vi "p33 operadoresf.vi"() -> ()   [LabVIEW 2017]
panel:
  in  "Enum 2":T1(ring)
  in  "path to BMP file":path
  in  "Tab Control":enum32{"Page 1"}(tab)
  out "2D Picture 15":picture
  out "2D Picture 16":picture
  in  "Slide 6":cluster{dbl, dbl, dbl, dbl, dbl}(slide)={0.0, 36.63140311804009, 185.40268456375838, 170.28523489932886, 152.88590604026845} scale=0.0..255.0
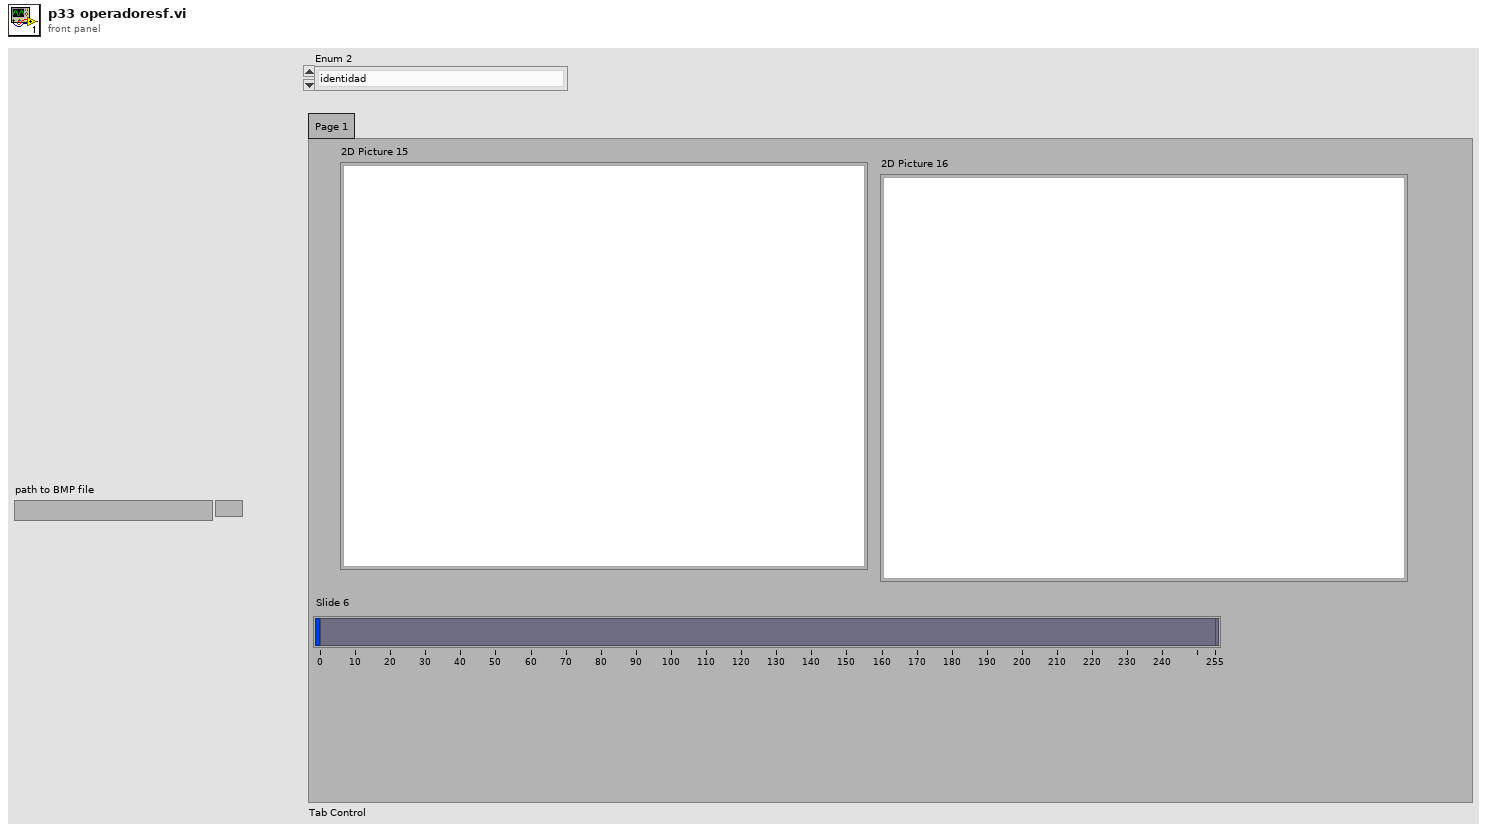
[diagram p1: front panel]
types:
  T1 = enum16{"identidad", "inverso o negativo", "umbral", "intervalo de umbral binario", "intervalo de umbral binario invertido", "umbral de la escala de grises", "umbral de la escala de grises invertido", "extension", "reduccion de nivel de gris", "ondulacion"}
  T2 = typedef "imagedata.ctl" = cluster{"image type":i32, "image depth":i32, "image":u8[], "mask":u8[], "colors":u32[], "Rectangle":cluster{"left":i16, "top":i16, "right":i16, "bottom":i16}}
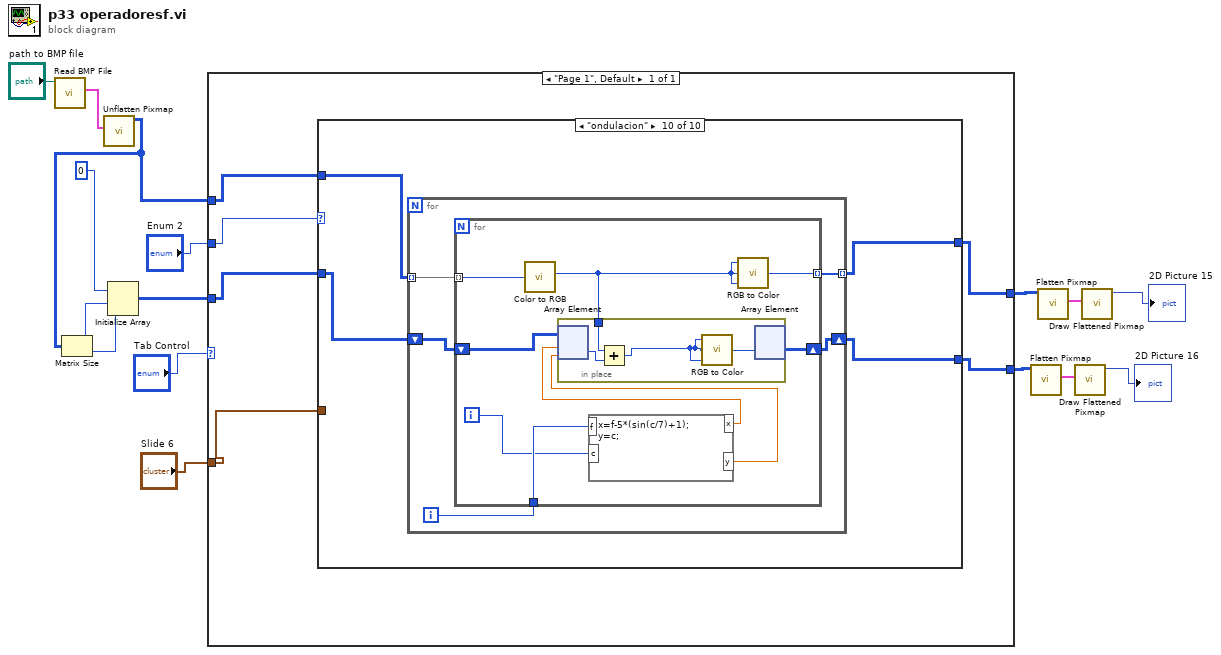
[diagram p0: block diagram]
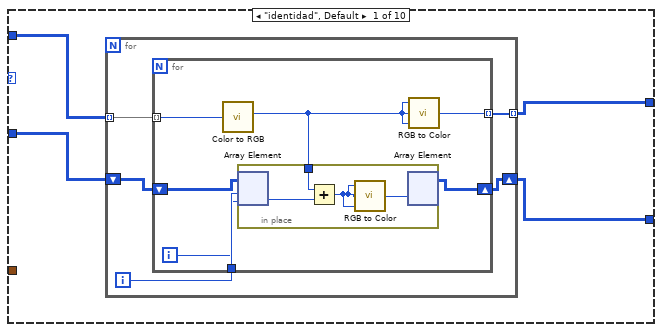
[diagram p2: hidden frame]
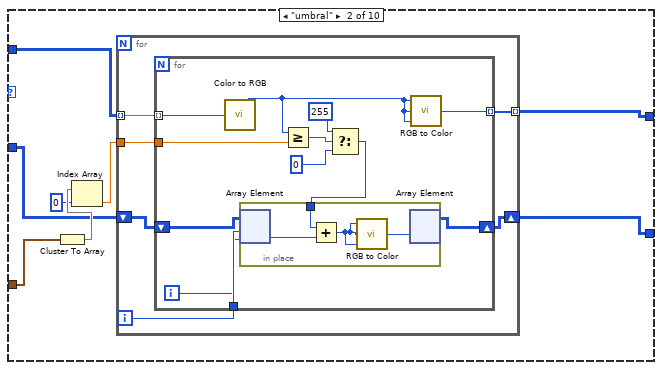
[diagram p3: hidden frame]
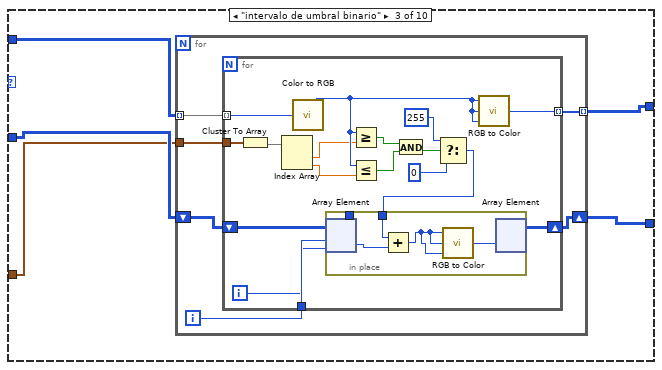
[diagram p4: hidden frame]
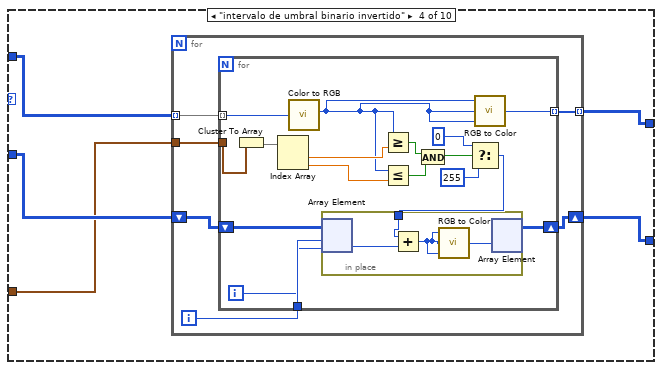
[diagram p5: hidden frame]
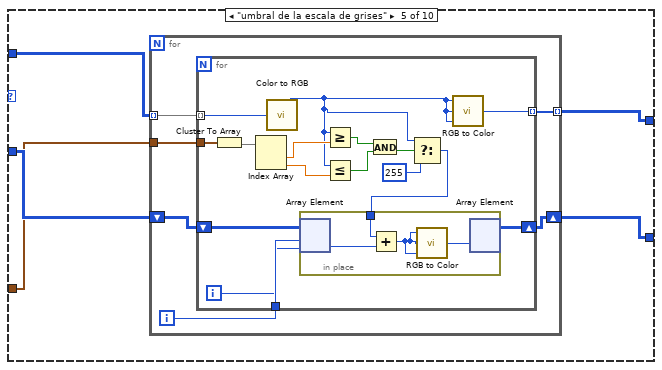
[diagram p6: hidden frame]
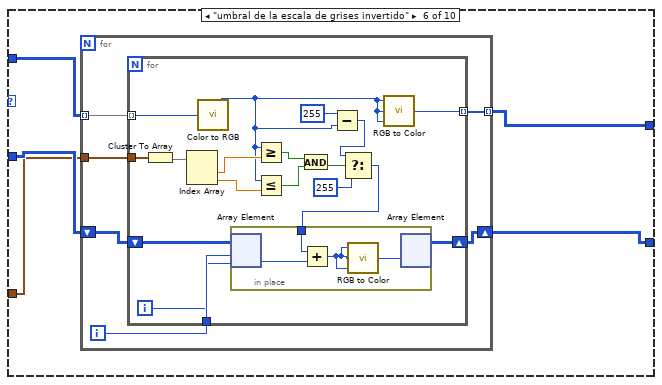
[diagram p7: hidden frame]
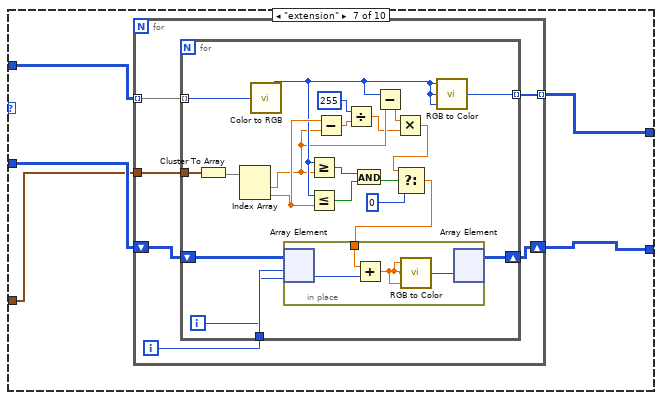
[diagram p8: hidden frame]
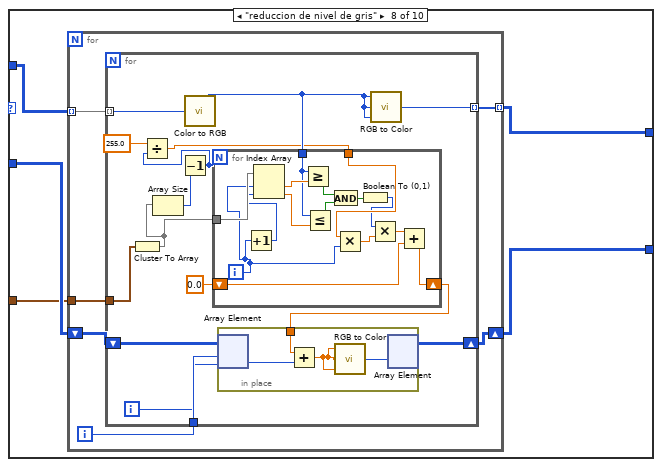
[diagram p9: hidden frame]
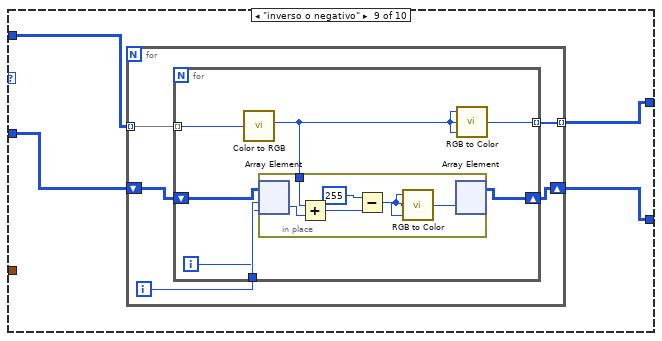
[diagram p10: hidden frame]
diagram:
  n1 = call <vilib>:"Read BMP File.vi"("path to BMP file"="path to BMP file") -> ("image data"=w15:T2)  [unwired: 8 in, 2 out]
  n2 = call <vilib>:"Unflatten Pixmap.vi"("image data"=w15) -> ("24-bit pixmap"=w11:u32[][])  [unwired: 4 in, 6 out]
  n3 = Matrix Size(0:w11) -> (1:w13:i32, 2:w12:i32)
  n4 = Initialize Array(0, w13, w12) -> (w10:i32[][])
  n5 = case shown="\"Page 1\", Default" "Tab Control" {
    tunnel: w11 -> [w20]
    tunnel: w10 -> [w18]
    tunnel: "Slide 6" -> [w17]
    tunnel: [w21] -> w3
    tunnel: [w22] -> w2
    tunnel: "Enum 2" -> [w19]
    frame "Page 1", Default {
      n6 = case shown="\"ondulacion\"" w19 {
        tunnel: w20 -> [w26 w47 w74 w109 w138 w172 w205 w241 w283 w307]
        tunnel: w18 -> [w25 w46 w75 w108 w139 w171 w204 w240 w282 w306]
        tunnel: [w24 w45 w77 w107 w141 w170 w202 w239 w285 w305] -> w22
        tunnel: [w23 w44 w76 w106 w140 w169 w203 w238 w284 w304] -> w21
        tunnel: w17 -> [_ w43 w73 w105 w137 w168 w201 w237 _ _]
        frame "identidad", Default {
          n7 = for {
            tunnel: w26 -> [w31] mode=indexing
            shift-right: [w29] -> w23
            shift-left: w25 -> [w30]
            tunnel: [w28] -> w24 mode=indexing
            i -> [w27]
            n8 = for {
              tunnel: w31 -> [w38] mode=indexing
              shift-right: [w35] -> w29
              shift-left: w30 -> [w37]
              tunnel: [w34] -> w28 mode=indexing
              tunnel: w27 -> [w33]
              i -> [w32]
              n9 = call <vilib>:"Color to RGB.vi"("Color"=w38) -> ("R"=w36:u8)  [unwired: 3 out]
              n10 = in-place {
                in-place-border: w36 -> [w42]
                n11 = in-place-array #1(w37, w33, w32) -> (w41:i32)
                n12 = Add(x=w42, y=w41) -> (x+y=w40:i32)
                n13 = call <vilib>:"RGB to Color.vi"("B"=w40, "G"=w40, "R"=w40) -> ("Color"=w39:u32)
                n14 = in-place-array #1(w39) -> (w35:i32[][])  [unwired: 2 out]
              }
              n15 = call <vilib>:"RGB to Color.vi"("B"=w36, "G"=w36, "R"=w36) -> ("Color"=w34:u32)
            }
          }
        }
        frame "umbral" {
          n16 = Cluster To Array(cluster=w43) -> (array=w50:dbl[])
          n17 = Index Array(array=w50, index=0) -> (element=w48:dbl)
          n18 = for {
            tunnel: w47 -> [w56] mode=indexing
            shift-right: [w54] -> w44
            shift-left: w46 -> [w55]
            tunnel: [w53] -> w45 mode=indexing
            tunnel: w48 -> [w51]
            i -> [w52]
            n19 = for {
              tunnel: w56 -> [w68] mode=indexing
              shift-right: [w66] -> w54
              shift-left: w55 -> [w67]
              tunnel: [w65] -> w53 mode=indexing
              tunnel: w52 -> [w64]
              tunnel: w51 -> [w57]
              i -> [w63]
              n20 = call <vilib>:"Color to RGB.vi"("Color"=w68) -> ("R"=w62:u8)  [unwired: 3 out]
              n21 = Greater Or Equal?(x=w62, y=w57) -> (x >= y?=w61:bool)
              n22 = Select(t=255, s=w61, f=0) -> (s? t:f=w58:i32)
              n23 = in-place {
                in-place-border: w58 -> [w72]
                n24 = in-place-array #2(w67, w64, w63) -> (w71:i32)
                n25 = Add(x=w72, y=w71) -> (x+y=w70:i32)
                n26 = call <vilib>:"RGB to Color.vi"("B"=w70, "G"=w70, "R"=w70) -> ("Color"=w69:u32)
                n27 = in-place-array #2(w69) -> (w66:i32[][])  [unwired: 2 out]
              }
              n28 = call <vilib>:"RGB to Color.vi"("B"=w62, "G"=w62, "R"=w62) -> ("Color"=w65:u32)
            }
          }
        }
        frame "intervalo de umbral binario" {
          n29 = for {
            tunnel: w74 -> [w83] mode=indexing
            shift-right: [w81] -> w76
            shift-left: w75 -> [w82]
            tunnel: [w80] -> w77 mode=indexing
            tunnel: w73 -> [w78]
            i -> [w79]
            n30 = for {
              tunnel: w83 -> [w100] mode=indexing
              shift-right: [w98] -> w81
              shift-left: w82 -> [w99]
              tunnel: [w97] -> w80 mode=indexing
              tunnel: w79 -> [w96]
              tunnel: w78 -> [w87]
              i -> [w95]
              n31 = Cluster To Array(cluster=w87) -> (array=w94:dbl[])
              n32 = Index Array(array=w94) -> (element #1=w86:dbl, element #2=w85:dbl)  [unwired: 2 in]
              n33 = call <vilib>:"Color to RGB.vi"("Color"=w100) -> ("R"=w92:u8)  [unwired: 3 out]
              n34 = Greater Or Equal?(x=w92, y=w86) -> (x >= y?=w93:bool)
              n35 = Less Or Equal?(x=w92, y=w85) -> (x <= y?=w91:bool)
              n36 = And(x=w93, y=w91) -> (x .and. y?=w90:bool)
              n37 = Select(t=255, s=w90, f=0) -> (s? t:f=w84:i32)
              n38 = in-place {
                in-place-border: [w102] -> _
                in-place-border: w84 -> [w103]
                n39 = in-place-array #3(w99, w96, w95) -> (w102:i32)
                n40 = Add(x=w103, y=w102) -> (x+y=w101:i32)
                n41 = call <vilib>:"RGB to Color.vi"("B"=w101, "G"=w101, "R"=w101) -> ("Color"=w104:u32)
                n42 = in-place-array #3(w104) -> (w98:i32[][])  [unwired: 2 out]
              }
              n43 = call <vilib>:"RGB to Color.vi"("B"=w92, "G"=w92, "R"=w92) -> ("Color"=w97:u32)
            }
          }
        }
        frame "intervalo de umbral binario invertido" {
          n44 = for {
            tunnel: w109 -> [w115] mode=indexing
            shift-right: [w113] -> w106
            shift-left: w108 -> [w114]
            tunnel: [w112] -> w107 mode=indexing
            tunnel: w105 -> [w110]
            i -> [w111]
            n45 = for {
              tunnel: w115 -> [w132] mode=indexing
              shift-right: [w130] -> w113
              shift-left: w114 -> [w131]
              tunnel: [w129] -> w112 mode=indexing
              tunnel: w111 -> [w128]
              tunnel: w110 -> [w126]
              i -> [w127]
              n46 = Cluster To Array(cluster=w126) -> (array=w125:dbl[])
              n47 = Index Array(array=w125) -> (element #1=w120:dbl, element #2=w118:dbl)  [unwired: 2 in]
              n48 = call <vilib>:"Color to RGB.vi"("Color"=w132) -> ("R"=w119:u8)  [unwired: 3 out]
              n49 = Greater Or Equal?(x=w119, y=w120) -> (x >= y?=w124:bool)
              n50 = Less Or Equal?(x=w119, y=w118) -> (x <= y?=w123:bool)
              n51 = And(x=w124, y=w123) -> (x .and. y?=w122:bool)
              n52 = Select(t=0, s=w122, f=255) -> (s? t:f=w116:i32)
              n53 = in-place {
                in-place-border: w116 -> [w133]
                n54 = in-place-array #4(w131, w128, w127) -> (w136:i32)
                n55 = Add(x=w133, y=w136) -> (x+y=w135:i32)
                n56 = call <vilib>:"RGB to Color.vi"("B"=w135, "G"=w135, "R"=w135) -> ("Color"=w134:u32)
                n57 = in-place-array #4(w134) -> (w130:i32[][])  [unwired: 2 out]
              }
              n58 = call <vilib>:"RGB to Color.vi"("B"=w119, "G"=w119, "R"=w119) -> ("Color"=w129:u32)
            }
          }
        }
        frame "umbral de la escala de grises" {
          n59 = for {
            tunnel: w138 -> [w147] mode=indexing
            shift-right: [w145] -> w140
            shift-left: w139 -> [w146]
            tunnel: [w144] -> w141 mode=indexing
            tunnel: w137 -> [w142]
            i -> [w143]
            n60 = for {
              tunnel: w147 -> [w163] mode=indexing
              shift-right: [w161] -> w145
              shift-left: w146 -> [w162]
              tunnel: [w160] -> w144 mode=indexing
              tunnel: w143 -> [w159]
              tunnel: w142 -> [w157]
              i -> [w158]
              n61 = Cluster To Array(cluster=w157) -> (array=w156:dbl[])
              n62 = Index Array(array=w156) -> (element #1=w155:dbl, element #2=w153:dbl)  [unwired: 2 in]
              n63 = call <vilib>:"Color to RGB.vi"("Color"=w163) -> ("R"=w148:u8)  [unwired: 3 out]
              n64 = Greater Or Equal?(x=w148, y=w155) -> (x >= y?=w154:bool)
              n65 = Less Or Equal?(x=w148, y=w153) -> (x <= y?=w152:bool)
              n66 = And(x=w154, y=w152) -> (x .and. y?=w151:bool)
              n67 = Select(t=w148, s=w151, f=255) -> (s? t:f=w149:i32)
              n68 = in-place {
                in-place-border: w149 -> [w164]
                n69 = in-place-array #5(w162, w159, w158) -> (w167:i32)
                n70 = Add(x=w164, y=w167) -> (x+y=w166:i32)
                n71 = call <vilib>:"RGB to Color.vi"("B"=w166, "G"=w166, "R"=w166) -> ("Color"=w165:u32)
                n72 = in-place-array #5(w165) -> (w161:i32[][])  [unwired: 2 out]
              }
              n73 = call <vilib>:"RGB to Color.vi"("B"=w148, "G"=w148, "R"=w148) -> ("Color"=w160:u32)
            }
          }
        }
        frame "umbral de la escala de grises invertido" {
          n74 = for {
            tunnel: w172 -> [w178] mode=indexing
            shift-right: [w176] -> w169
            shift-left: w171 -> [w177]
            tunnel: [w175] -> w170 mode=indexing
            tunnel: w168 -> [w173]
            i -> [w174]
            n75 = for {
              tunnel: w178 -> [w196] mode=indexing
              shift-right: [w194] -> w176
              shift-left: w177 -> [w195]
              tunnel: [w193] -> w175 mode=indexing
              tunnel: w174 -> [w192]
              tunnel: w173 -> [w190]
              i -> [w191]
              n76 = Cluster To Array(cluster=w190) -> (array=w189:dbl[])
              n77 = Index Array(array=w189) -> (element #1=w188:dbl, element #2=w186:dbl)  [unwired: 2 in]
              n78 = call <vilib>:"Color to RGB.vi"("Color"=w196) -> ("R"=w180:u8)  [unwired: 3 out]
              n79 = Greater Or Equal?(x=w180, y=w188) -> (x >= y?=w187:bool)
              n80 = Less Or Equal?(x=w180, y=w186) -> (x <= y?=w185:bool)
              n81 = And(x=w187, y=w185) -> (x .and. y?=w184:bool)
              n82 = Subtract(x=255, y=w180) -> (x-y=w179:i32)
              n83 = Select(t=w179, s=w184, f=255) -> (s? t:f=w182:i32)
              n84 = in-place {
                in-place-border: w182 -> [w197]
                n85 = in-place-array #6(w195, w192, w191) -> (w200:i32)
                n86 = Add(x=w197, y=w200) -> (x+y=w199:i32)
                n87 = call <vilib>:"RGB to Color.vi"("B"=w199, "G"=w199, "R"=w199) -> ("Color"=w198:u32)
                n88 = in-place-array #6(w198) -> (w194:i32[][])  [unwired: 2 out]
              }
              n89 = call <vilib>:"RGB to Color.vi"("B"=w180, "G"=w180, "R"=w180) -> ("Color"=w193:u32)
            }
          }
        }
        frame "extension" {
          n90 = for {
            tunnel: w205 -> [w211] mode=indexing
            shift-right: [w209] -> w203
            shift-left: w204 -> [w210]
            tunnel: [w208] -> w202 mode=indexing
            tunnel: w201 -> [w206]
            i -> [w207]
            n91 = for {
              tunnel: w211 -> [w232] mode=indexing
              shift-right: [w230] -> w209
              shift-left: w210 -> [w231]
              tunnel: [w229] -> w208 mode=indexing
              tunnel: w207 -> [w228]
              tunnel: w206 -> [w226]
              i -> [w227]
              n92 = Cluster To Array(cluster=w226) -> (array=w225:dbl[])
              n93 = Index Array(array=w225) -> (element #1=w216:dbl, element #2=w220:dbl)  [unwired: 2 in]
              n94 = call <vilib>:"Color to RGB.vi"("Color"=w232) -> ("R"=w217:u8)  [unwired: 3 out]
              n95 = Greater Or Equal?(x=w217, y=w216) -> (x >= y?=w224:bool)
              n96 = Less Or Equal?(x=w217, y=w220) -> (x <= y?=w223:bool)
              n97 = Subtract(x=w220, y=w216) -> (x-y=w219:dbl)
              n98 = Divide(x=255, y=w219) -> (x/y=w214:dbl)
              n99 = And(x=w224, y=w223) -> (x .and. y?=w222:bool)
              n100 = Subtract(x=w217, y=w216) -> (x-y=w215:dbl)
              n101 = Multiply(x=w215, y=w214) -> (x*y=w213:dbl)
              n102 = Select(t=w213, s=w222, f=0) -> (s? t:f=w212:dbl)
              n103 = in-place {
                in-place-border: w212 -> [w233]
                n104 = in-place-array #7(w231, w228, w227) -> (w236:i32)
                n105 = Add(x=w233, y=w236) -> (x+y=w235:dbl)
                n106 = call <vilib>:"RGB to Color.vi"("B"=w235, "G"=w235, "R"=w235) -> ("Color"=w234:u32)
                n107 = in-place-array #7(w234) -> (w230:i32[][])  [unwired: 2 out]
              }
              n108 = call <vilib>:"RGB to Color.vi"("B"=w217, "G"=w217, "R"=w217) -> ("Color"=w229:u32)
            }
          }
        }
        frame "reduccion de nivel de gris" {
          n109 = for {
            tunnel: w241 -> [w247] mode=indexing
            shift-right: [w245] -> w238
            shift-left: w240 -> [w246]
            tunnel: [w244] -> w239 mode=indexing
            tunnel: w237 -> [w242]
            i -> [w243]
            n110 = for {
              tunnel: w247 -> [w262] mode=indexing
              shift-right: [w260] -> w245
              shift-left: w246 -> [w261]
              tunnel: [w259] -> w244 mode=indexing
              tunnel: w243 -> [w258]
              tunnel: w242 -> [w248]
              i -> [w257]
              n111 = Cluster To Array(cluster=w248) -> (array=w255:dbl[])
              n112 = Array Size(array=w255) -> (size(s)=w256:i32)
              n113 = Decrement(x=w256) -> (x-1=w252:i32)
              n114 = Divide(x=255.0, y=w252) -> (x/y=w251:dbl)
              n115 = call <vilib>:"Color to RGB.vi"("Color"=w262) -> ("R"=w254:u8)  [unwired: 3 out]
              n116 = for {
                N: w252 -> [_]
                tunnel: w255 -> [w277]
                tunnel: w254 -> [w274]
                tunnel: w251 -> [w269]
                shift-right: [w263] -> w249
                shift-left: 0.0 -> [w264]
                i -> [w268]
                n117 = Increment(x=w268) -> (x+1=w276:i32)
                n118 = Index Array(array=w277, index #1=w268, index #2=w276) -> (element #1=w275:dbl, element #2=w273:dbl)
                n119 = Greater Or Equal?(x=w274, y=w275) -> (x >= y?=w271:bool)
                n120 = Less Or Equal?(x=w274, y=w273) -> (x <= y?=w272:bool)
                n121 = And(x=w271, y=w272) -> (x .and. y?=w270:bool)
                n122 = Multiply(x=w269, y=w268) -> (x*y=w265:dbl)
                n123 = Boolean To (0,1)(Boolean=w270) -> (0, 1=w266:i16)
                n124 = Multiply(x=w266, y=w265) -> (x*y=w267:dbl)
                n125 = Add(x=w267, y=w264) -> (x+y=w263:dbl)
              }
              n126 = in-place {
                in-place-border: w249 -> [w278]
                n127 = in-place-array #8(w261, w258, w257) -> (w281:i32)
                n128 = Add(x=w278, y=w281) -> (x+y=w280:dbl)
                n129 = call <vilib>:"RGB to Color.vi"("B"=w280, "G"=w280, "R"=w280) -> ("Color"=w279:u32)
                n130 = in-place-array #8(w279) -> (w260:i32[][])  [unwired: 2 out]
              }
              n131 = call <vilib>:"RGB to Color.vi"("B"=w254, "G"=w254, "R"=w254) -> ("Color"=w259:u32)
            }
          }
        }
        frame "inverso o negativo" {
          n132 = for {
            tunnel: w283 -> [w290] mode=indexing
            shift-right: [w288] -> w284
            shift-left: w282 -> [w289]
            tunnel: [w287] -> w285 mode=indexing
            i -> [w286]
            n133 = for {
              tunnel: w290 -> [w297] mode=indexing
              shift-right: [w295] -> w288
              shift-left: w289 -> [w296]
              tunnel: [w294] -> w287 mode=indexing
              tunnel: w286 -> [w293]
              i -> [w292]
              n134 = call <vilib>:"Color to RGB.vi"("Color"=w297) -> ("R"=w291:u8)  [unwired: 3 out]
              n135 = in-place {
                in-place-border: w291 -> [w300]
                n136 = in-place-array #9(w296, w293, w292) -> (w299:i32)
                n137 = Add(x=w300, y=w299) -> (x+y=w298:i32)
                n138 = Subtract(x=u8 255, y=w298) -> (x-y=w301:i32)
                n139 = call <vilib>:"RGB to Color.vi"("B"=w301, "G"=w301, "R"=w301) -> ("Color"=w303:u32)
                n140 = in-place-array #9(w303) -> (w295:i32[][])  [unwired: 2 out]
              }
              n141 = call <vilib>:"RGB to Color.vi"("B"=w291, "G"=w291, "R"=w291) -> ("Color"=w294:u32)
            }
          }
        }
        frame "ondulacion" {
          n142 = for {
            tunnel: w307 -> [w312] mode=indexing
            shift-right: [w310] -> w304
            shift-left: w306 -> [w311]
            tunnel: [w309] -> w305 mode=indexing
            i -> [w308]
            n143 = for {
              tunnel: w312 -> [w321] mode=indexing
              shift-right: [w319] -> w310
              shift-left: w311 -> [w320]
              tunnel: [w318] -> w309 mode=indexing
              tunnel: w308 -> [w316]
              i -> [w315]
              n144 = call <vilib>:"Color to RGB.vi"("Color"=w321) -> ("R"=w317:u8)  [unwired: 3 out]
              n145 = formula code="x=f-5*(sin(c/7)+1);\ny=c;"("f"=w316, "c"=w315) -> ("x"=w314:dbl, "y"=w313:dbl)
              n146 = in-place {
                in-place-border: w317 -> [w324]
                n147 = in-place-array #10(w320, w314, w313) -> (w323:i32)
                n148 = Add(x=w324, y=w323) -> (x+y=w322:i32)
                n149 = call <vilib>:"RGB to Color.vi"("B"=w322, "G"=w322, "R"=w322) -> ("Color"=w325:u32)
                n150 = in-place-array #10(w325) -> (w319:i32[][])  [unwired: 2 out]
              }
              n151 = call <vilib>:"RGB to Color.vi"("B"=w317, "G"=w317, "R"=w317) -> ("Color"=w318:u32)
            }
          }
        }
      }
    }
  }
  n152 = call <vilib>:"Flatten Pixmap.vi"("24-bit pixmap"=w3) -> ("image data"=w4:T2)  [unwired: 10 in]
  n153 = call <vilib>:"Flatten Pixmap.vi"("24-bit pixmap"=w2) -> ("image data"=w5:T2)  [unwired: 10 in]
  n154 = call <vilib>:"Draw Flattened Pixmap.vi"("image data"=w4) -> ("new picture"=→"2D Picture 16":picture)  [unwired: 8 in]
  n155 = call <vilib>:"Draw Flattened Pixmap.vi"("image data"=w5) -> ("new picture"=→"2D Picture 15":picture)  [unwired: 8 in]
